vi "Восстановление мишеней (SubVI).vi"(2 "error in":errorcluster, 7 "Параметры всех мишеней":T1, 13 "Кластер reference":T2) -> (15 "error out":errorcluster)   [LabVIEW 2013]
doc: "Восстановление размеров и позиций мишеней"
panel:
  out "М10":refnum<vi>
  out "М9":refnum<vi>
  out "М8":refnum<vi>
  out "М7":refnum<vi>
  out "М6":refnum<vi>
  out "М5":refnum<vi>
  out "М4":refnum<vi>
  out "М3":refnum<vi>
  out "М2":refnum<vi>
  out "М1":refnum<vi>
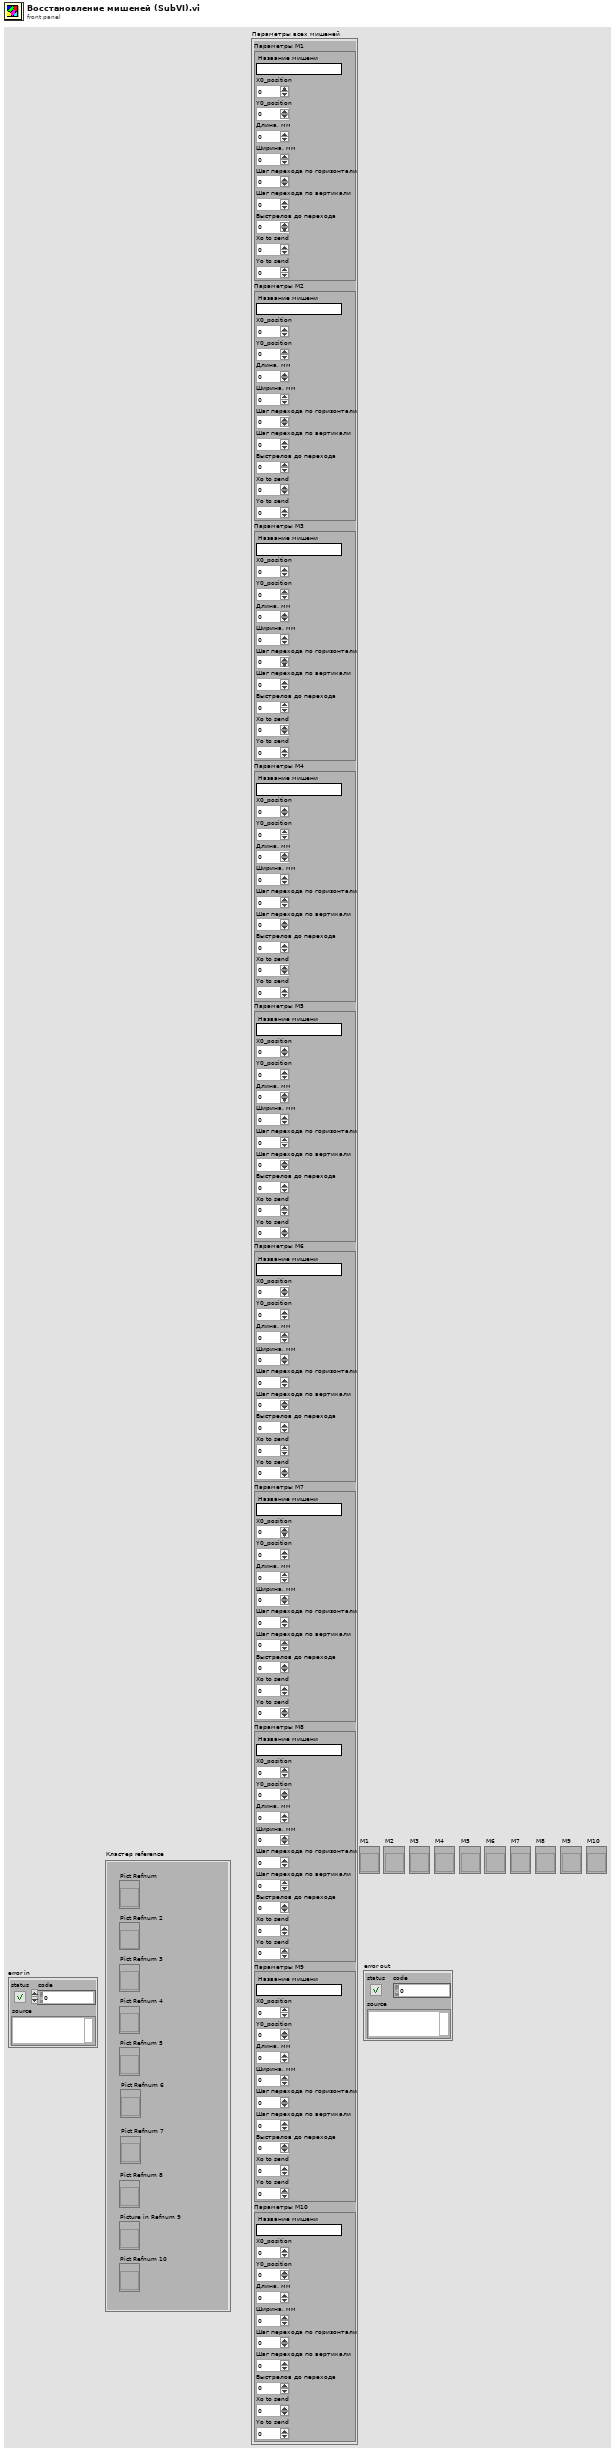
[diagram p1: front panel]
types:
  T1 = cluster{"Параметры М1":cluster{"Название мишени":string, "Х0_position":u16, "Y0_position":u16, "Длина, мм":u16, "Ширина, мм":u16, "Шаг перехода по горизонтали":dbl, "Шаг перехода по вертикали":dbl, "Выстрелов до перехода":u16, "Xo to send ":u16, "Yo to send":u16}, "Параметры М2":cluster{"Название мишени":string, "Х0_position":u16, "Y0_position":u16, "Длина, мм":u16, "Ширина, мм":u16, "Шаг перехода по горизонтали":dbl, "Шаг перехода по вертикали":dbl, "Выстрелов до перехода":u16, "Xo to send ":u16, "Yo to send":u16}, "Параметры М3":cluster{"Название мишени":string, "Х0_position":u16, "Y0_position":u16, "Длина, мм":u16, "Ширина, мм":u16, "Шаг перехода по горизонтали":dbl, "Шаг перехода по вертикали":dbl, "Выстрелов до перехода":u16, "Xo to send ":u16, "Yo to send":u16}, "Параметры М4":cluster{"Название мишени":string, "Х0_position":u16, "Y0_position":u16, "Длина, мм":u16, "Ширина, мм":u16, "Шаг перехода по горизонтали":dbl, "Шаг перехода по вертикали":dbl, "Выстрелов до перехода":u16, "Xo to send ":u16, "Yo to send":u16}, "Параметры М5":cluster{"Название мишени":string, "Х0_position":u16, "Y0_position":u16, "Длина, мм":u16, "Ширина, мм":u16, "Шаг перехода по горизонтали":dbl, "Шаг перехода по вертикали":dbl, "Выстрелов до перехода":u16, "Xo to send ":u16, "Yo to send":u16}, "Параметры М6":cluster{"Название мишени":string, "Х0_position":u16, "Y0_position":u16, "Длина, мм":u16, "Ширина, мм":u16, "Шаг перехода по горизонтали":dbl, "Шаг перехода по вертикали":dbl, "Выстрелов до перехода":u16, "Xo to send ":u16, "Yo to send":u16}, "Параметры М7":cluster{"Название мишени":string, "Х0_position":u16, "Y0_position":u16, "Длина, мм":u16, "Ширина, мм":u16, "Шаг перехода по горизонтали":dbl, "Шаг перехода по вертикали":dbl, "Выстрелов до перехода":u16, "Xo to send ":u16, "Yo to send":u16}, "Параметры М8":cluster{"Название мишени":string, "Х0_position":u16, "Y0_position":u16, "Длина, мм":u16, "Ширина, мм":u16, "Шаг перехода по горизонтали":dbl, "Шаг перехода по вертикали":dbl, "Выстрелов до перехода":u16, "Xo to send ":u16, "Yo to send":u16}, "Параметры М9":cluster{"Название мишени":string, "Х0_position":u16, "Y0_position":u16, "Длина, мм":u16, "Ширина, мм":u16, "Шаг перехода по горизонтали":dbl, "Шаг перехода по вертикали":dbl, "Выстрелов до перехода":u16, "Xo to send ":u16, "Yo to send":u16}, "Параметры М10":cluster{"Название мишени":string, "Х0_position":u16, "Y0_position":u16, "Длина, мм":u16, "Ширина, мм":u16, "Шаг перехода по горизонтали":dbl, "Шаг перехода по вертикали":dbl, "Выстрелов до перехода":u16, "Xo to send ":u16, "Yo to send":u16}}
  T2 = cluster{"Pict Refnum":refnum<vi>, "Pict Refnum 2":refnum<vi>, "Pict Refnum 3":refnum<vi>, "Pict Refnum 4":refnum<vi>, "Pict Refnum 5":refnum<vi>, "Pict Refnum 6":refnum<vi>, "Pict Refnum 7":refnum<vi>, "Pict Refnum 8":refnum<vi>, "Picture in Refnum 9":refnum<vi>, "Pict Refnum 10":refnum<vi>}
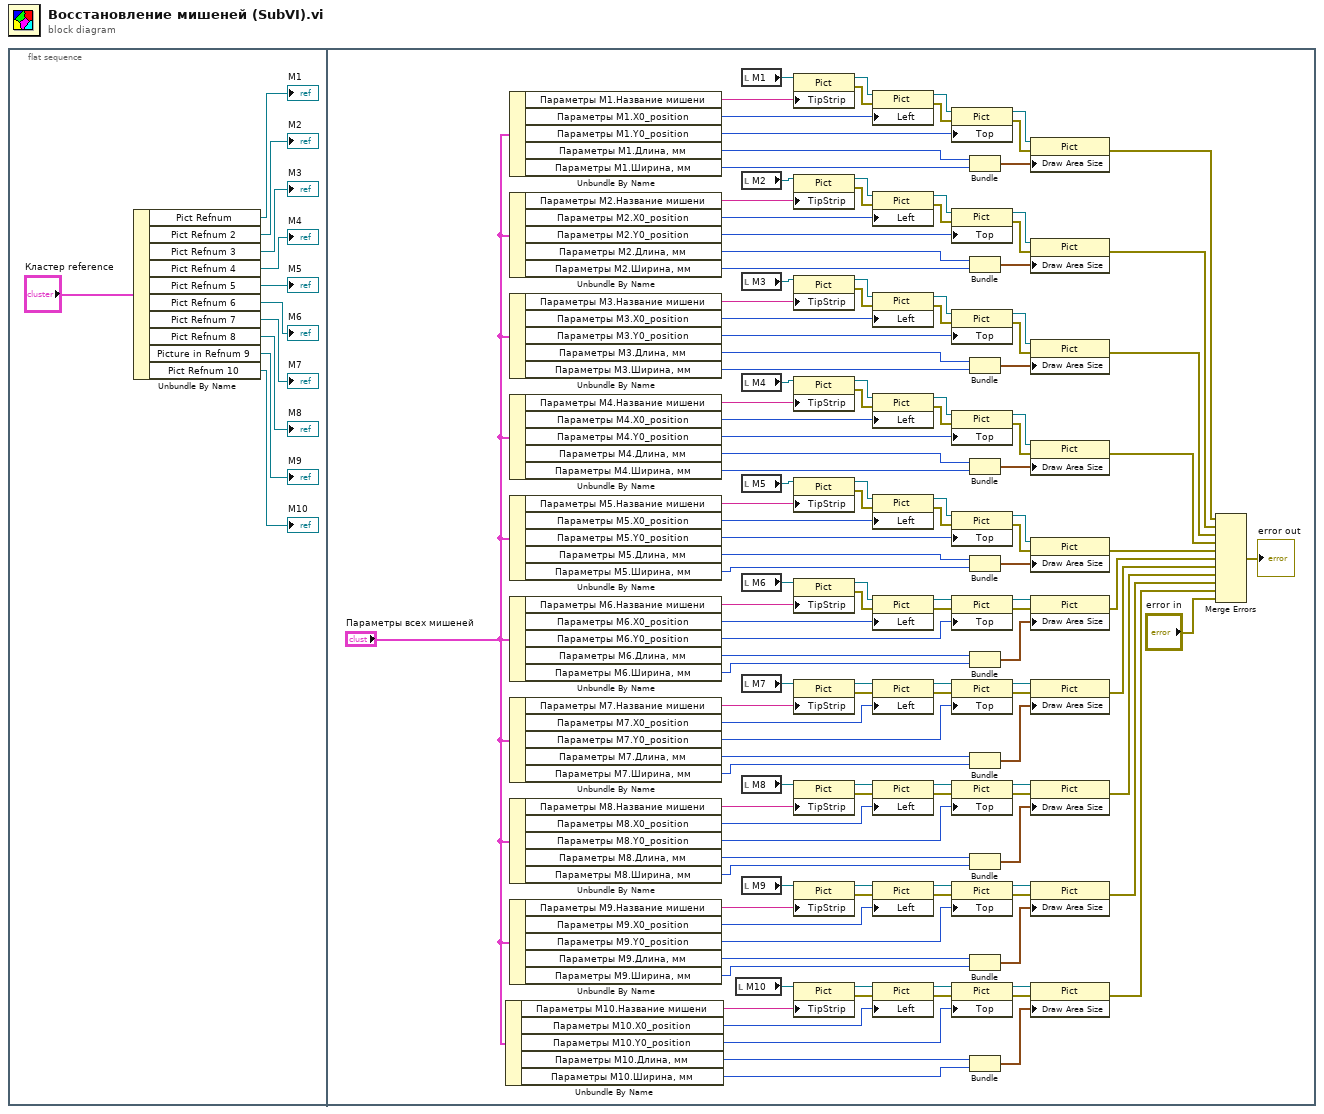
[diagram p0: block diagram]
diagram:
  n1 = flat-sequence {
    frame #0 {
      n2 = Unbundle By Name("Кластер reference") -> ("Pict Refnum"=→"М1":refnum<vi>, "Pict Refnum 2"=→"М2":refnum<vi>, "Pict Refnum 3"=→"М3":refnum<vi>, "Pict Refnum 4"=→"М4":refnum<vi>, "Pict Refnum 5"=→"М5":refnum<vi>, "Pict Refnum 6"=→"М6":refnum<vi>, "Pict Refnum 7"=→"М7":refnum<vi>, "Pict Refnum 8"=→"М8":refnum<vi>, "Picture in Refnum 9"=→"М9":refnum<vi>, "Pict Refnum 10"=→"М10":refnum<vi>)
    }
    frame #1 {
      n3 = Unbundle By Name("Параметры всех мишеней") -> ("Параметры М10.Название мишени"=w107:string, "Параметры М10.Х0_position"=w108:u16, "Параметры М10.Y0_position"=w109:u16, "Параметры М10.Длина, мм"=w110:u16, "Параметры М10.Ширина, мм"=w111:u16)
      n4 = Unbundle By Name("Параметры всех мишеней") -> ("Параметры М1.Название мишени"=w18:string, "Параметры М1.Х0_position"=w19:u16, "Параметры М1.Y0_position"=w20:u16, "Параметры М1.Длина, мм"=w14:u16, "Параметры М1.Ширина, мм"=w15:u16)
      n5 = Unbundle By Name("Параметры всех мишеней") -> ("Параметры М2.Название мишени"=w30:string, "Параметры М2.Х0_position"=w31:u16, "Параметры М2.Y0_position"=w32:u16, "Параметры М2.Длина, мм"=w16:u16, "Параметры М2.Ширина, мм"=w17:u16)
      n6 = Unbundle By Name("Параметры всех мишеней") -> ("Параметры М3.Название мишени"=w40:string, "Параметры М3.Х0_position"=w41:u16, "Параметры М3.Y0_position"=w42:u16, "Параметры М3.Длина, мм"=w37:u16, "Параметры М3.Ширина, мм"=w38:u16)
      n7 = Unbundle By Name("Параметры всех мишеней") -> ("Параметры М4.Название мишени"=w58:string, "Параметры М4.Х0_position"=w59:u16, "Параметры М4.Y0_position"=w60:u16, "Параметры М4.Длина, мм"=w55:u16, "Параметры М4.Ширина, мм"=w56:u16)
      n8 = Unbundle By Name("Параметры всех мишеней") -> ("Параметры М5.Название мишени"=w61:string, "Параметры М5.Х0_position"=w62:u16, "Параметры М5.Y0_position"=w63:u16, "Параметры М5.Длина, мм"=w64:u16, "Параметры М5.Ширина, мм"=w65:u16)
      n9 = Unbundle By Name("Параметры всех мишеней") -> ("Параметры М6.Название мишени"=w67:string, "Параметры М6.Х0_position"=w68:u16, "Параметры М6.Y0_position"=w69:u16, "Параметры М6.Длина, мм"=w70:u16, "Параметры М6.Ширина, мм"=w71:u16)
      n10 = Unbundle By Name("Параметры всех мишеней") -> ("Параметры М7.Название мишени"=w92:string, "Параметры М7.Х0_position"=w93:u16, "Параметры М7.Y0_position"=w94:u16, "Параметры М7.Длина, мм"=w90:u16, "Параметры М7.Ширина, мм"=w91:u16)
      n11 = Unbundle By Name("Параметры всех мишеней") -> ("Параметры М8.Название мишени"=w95:string, "Параметры М8.Х0_position"=w96:u16, "Параметры М8.Y0_position"=w97:u16, "Параметры М8.Длина, мм"=w98:u16, "Параметры М8.Ширина, мм"=w99:u16)
      n12 = Unbundle By Name("Параметры всех мишеней") -> ("Параметры М9.Название мишени"=w101:string, "Параметры М9.Х0_position"=w102:u16, "Параметры М9.Y0_position"=w103:u16, "Параметры М9.Длина, мм"=w104:u16, "Параметры М9.Ширина, мм"=w105:u16)
      n13 = local read "М10"() -> (w76:refnum<vi>)
      n14 = local read "М1"() -> (w27:refnum<vi>)
      n15 = local read "М2"() -> (w28:refnum<vi>)
      n16 = local read "М3"() -> (w33:refnum<vi>)
      n17 = local read "М4"() -> (w48:refnum<vi>)
      n18 = local read "М5"() -> (w47:refnum<vi>)
      n19 = local read "М6"() -> (w46:refnum<vi>)
      n20 = local read "М7"() -> (w82:refnum<vi>)
      n21 = local read "М8"() -> (w81:refnum<vi>)
      n22 = local read "М9"() -> (w80:refnum<vi>)
      n23 = property on="Property Node" class="Pict"(reference=w27, "TipStrip"=w18) -> (reference out=w13:refnum<vi>, error out=w113:errorcluster)  [unwired: 1 in]
      n24 = property on="Property Node" class="Pict"(reference=w28, "TipStrip"=w30) -> (reference out=w26:refnum<vi>, error out=w116:errorcluster)  [unwired: 1 in]
      n25 = property on="Property Node" class="Pict"(reference=w33, "TipStrip"=w40) -> (reference out=w34:refnum<vi>, error out=w119:errorcluster)  [unwired: 1 in]
      n26 = property on="Property Node" class="Pict"(reference=w48, "TipStrip"=w58) -> (reference out=w54:refnum<vi>, error out=w122:errorcluster)  [unwired: 1 in]
      n27 = property on="Property Node" class="Pict"(reference=w47, "TipStrip"=w61) -> (reference out=w49:refnum<vi>, error out=w125:errorcluster)  [unwired: 1 in]
      n28 = property on="Property Node" class="Pict"(reference=w46, "TipStrip"=w67) -> (reference out=w45:refnum<vi>, error out=w128:errorcluster)  [unwired: 1 in]
      n29 = property on="Property Node" class="Pict"(reference=w82, "TipStrip"=w92) -> (reference out=w88:refnum<vi>, error out=w131:errorcluster)  [unwired: 1 in]
      n30 = property on="Property Node" class="Pict"(reference=w81, "TipStrip"=w95) -> (reference out=w83:refnum<vi>, error out=w134:errorcluster)  [unwired: 1 in]
      n31 = property on="Property Node" class="Pict"(reference=w80, "TipStrip"=w101) -> (reference out=w79:refnum<vi>, error out=w137:errorcluster)  [unwired: 1 in]
      n32 = property on="Property Node" class="Pict"(reference=w76, "TipStrip"=w107) -> (reference out=w73:refnum<vi>, error out=w140:errorcluster)  [unwired: 1 in]
      n33 = property on="Property Node" class="Pict"(reference=w13, error in=w113, "Left"=w19) -> (reference out=w22:refnum<vi>, error out=w114:errorcluster)
      n34 = property on="Property Node" class="Pict"(reference=w26, error in=w116, "Left"=w31) -> (reference out=w25:refnum<vi>, error out=w117:errorcluster)
      n35 = property on="Property Node" class="Pict"(reference=w34, error in=w119, "Left"=w41) -> (reference out=w35:refnum<vi>, error out=w120:errorcluster)
      n36 = property on="Property Node" class="Pict"(reference=w54, error in=w122, "Left"=w59) -> (reference out=w53:refnum<vi>, error out=w123:errorcluster)
      n37 = property on="Property Node" class="Pict"(reference=w49, error in=w125, "Left"=w62) -> (reference out=w50:refnum<vi>, error out=w126:errorcluster)
      n38 = property on="Property Node" class="Pict"(reference=w45, error in=w128, "Left"=w68) -> (reference out=w44:refnum<vi>, error out=w129:errorcluster)
      n39 = property on="Property Node" class="Pict"(reference=w88, error in=w131, "Left"=w93) -> (reference out=w87:refnum<vi>, error out=w132:errorcluster)
      n40 = property on="Property Node" class="Pict"(reference=w83, error in=w134, "Left"=w96) -> (reference out=w84:refnum<vi>, error out=w135:errorcluster)
      n41 = property on="Property Node" class="Pict"(reference=w79, error in=w137, "Left"=w102) -> (reference out=w78:refnum<vi>, error out=w138:errorcluster)
      n42 = property on="Property Node" class="Pict"(reference=w73, error in=w140, "Left"=w108) -> (reference out=w74:refnum<vi>, error out=w141:errorcluster)
      n43 = property on="Property Node" class="Pict"(reference=w22, error in=w114, "Top"=w20) -> (reference out=w23:refnum<vi>, error out=w115:errorcluster)
      n44 = property on="Property Node" class="Pict"(reference=w25, error in=w117, "Top"=w32) -> (reference out=w24:refnum<vi>, error out=w118:errorcluster)
      n45 = property on="Property Node" class="Pict"(reference=w35, error in=w120, "Top"=w42) -> (reference out=w36:refnum<vi>, error out=w121:errorcluster)
      n46 = property on="Property Node" class="Pict"(reference=w53, error in=w123, "Top"=w60) -> (reference out=w52:refnum<vi>, error out=w124:errorcluster)
      n47 = property on="Property Node" class="Pict"(reference=w50, error in=w126, "Top"=w63) -> (reference out=w51:refnum<vi>, error out=w127:errorcluster)
      n48 = property on="Property Node" class="Pict"(reference=w44, error in=w129, "Top"=w69) -> (reference out=w43:refnum<vi>, error out=w130:errorcluster)
      n49 = property on="Property Node" class="Pict"(reference=w87, error in=w132, "Top"=w94) -> (reference out=w86:refnum<vi>, error out=w133:errorcluster)
      n50 = property on="Property Node" class="Pict"(reference=w84, error in=w135, "Top"=w97) -> (reference out=w85:refnum<vi>, error out=w136:errorcluster)
      n51 = property on="Property Node" class="Pict"(reference=w78, error in=w138, "Top"=w103) -> (reference out=w77:refnum<vi>, error out=w139:errorcluster)
      n52 = property on="Property Node" class="Pict"(reference=w74, error in=w141, "Top"=w109) -> (reference out=w75:refnum<vi>, error out=w142:errorcluster)
      n53 = Bundle("Длина, мм"=w14, "Ширина, мм"=w15) -> (w21:cluster{"Длина, мм":u16, "Ширина, мм":u16})  [unwired: 1 in]
      n54 = Bundle("Длина, мм"=w16, "Ширина, мм"=w17) -> (w29:cluster{"Длина, мм":u16, "Ширина, мм":u16})  [unwired: 1 in]
      n55 = Bundle("Длина, мм"=w37, "Ширина, мм"=w38) -> (w39:cluster{"Длина, мм":u16, "Ширина, мм":u16})  [unwired: 1 in]
      n56 = Bundle("Длина, мм"=w55, "Ширина, мм"=w56) -> (w57:cluster{"Длина, мм":u16, "Ширина, мм":u16})  [unwired: 1 in]
      n57 = Bundle("Длина, мм"=w64, "Ширина, мм"=w65) -> (w66:cluster{"Длина, мм":u16, "Ширина, мм":u16})  [unwired: 1 in]
      n58 = Bundle("Длина, мм"=w70, "Ширина, мм"=w71) -> (w72:cluster{"Длина, мм":u16, "Ширина, мм":u16})  [unwired: 1 in]
      n59 = Bundle("Длина, мм"=w90, "Ширина, мм"=w91) -> (w89:cluster{"Длина, мм":u16, "Ширина, мм":u16})  [unwired: 1 in]
      n60 = Bundle("Длина, мм"=w98, "Ширина, мм"=w99) -> (w100:cluster{"Длина, мм":u16, "Ширина, мм":u16})  [unwired: 1 in]
      n61 = Bundle("Длина, мм"=w104, "Ширина, мм"=w105) -> (w106:cluster{"Длина, мм":u16, "Ширина, мм":u16})  [unwired: 1 in]
      n62 = Bundle("Длина, мм"=w110, "Ширина, мм"=w111) -> (w112:cluster{"Длина, мм":u16, "Ширина, мм":u16})  [unwired: 1 in]
      n63 = property on="Property Node" class="Pict"(reference=w23, error in=w115, "Draw Area Size"=w21) -> (error out=w143:errorcluster)  [unwired: 1 out]
      n64 = property on="Property Node" class="Pict"(reference=w24, error in=w118, "Draw Area Size"=w29) -> (error out=w144:errorcluster)  [unwired: 1 out]
      n65 = property on="Property Node" class="Pict"(reference=w36, error in=w121, "Draw Area Size"=w39) -> (error out=w145:errorcluster)  [unwired: 1 out]
      n66 = property on="Property Node" class="Pict"(reference=w52, error in=w124, "Draw Area Size"=w57) -> (error out=w146:errorcluster)  [unwired: 1 out]
      n67 = property on="Property Node" class="Pict"(reference=w51, error in=w127, "Draw Area Size"=w66) -> (error out=w147:errorcluster)  [unwired: 1 out]
      n68 = property on="Property Node" class="Pict"(reference=w43, error in=w130, "Draw Area Size"=w72) -> (error out=w148:errorcluster)  [unwired: 1 out]
      n69 = property on="Property Node" class="Pict"(reference=w86, error in=w133, "Draw Area Size"=w89) -> (error out=w149:errorcluster)  [unwired: 1 out]
      n70 = property on="Property Node" class="Pict"(reference=w85, error in=w136, "Draw Area Size"=w100) -> (error out=w150:errorcluster)  [unwired: 1 out]
      n71 = property on="Property Node" class="Pict"(reference=w77, error in=w139, "Draw Area Size"=w106) -> (error out=w151:errorcluster)  [unwired: 1 out]
      n72 = property on="Property Node" class="Pict"(reference=w75, error in=w142, "Draw Area Size"=w112) -> (error out=w152:errorcluster)  [unwired: 1 out]
      n73 = Merge Errors(w143, w144, w145, w146, w147, w148, w149, w150, w151, w152, "error in") -> (→"error out":errorcluster)
    }
  }
